vi "Corr_coeff_array.vi"(2 "Sampling frequency":dbl format="%.2f", 3 "U2":dbl[](array[numeric]) format="%.2f", 4 "U1":dbl[](array[numeric]) format="%.2f", 5 "Slippage range":i32) -> (0 "Correlation Coefficient":dbl[](array[numeric]) format="%.2f", 1 "Time":dbl[](array[numeric]) format="%.2f")   [LabVIEW 2010]
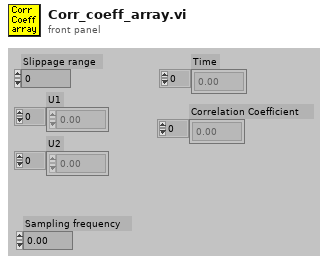
[diagram p1: front panel]
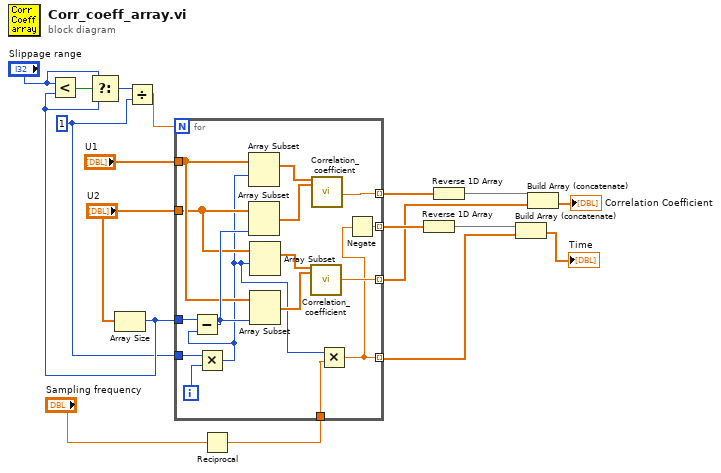
[diagram p0: block diagram]
diagram:
  w1 = 1 ("y")
  n1 = Array Size(array="U2") -> (size(s)=w7:i32)
  n2 = Less?(x="Slippage range", y=w7) -> (x < y?=w8:bool)
  n3 = Select(t="Slippage range", s=w8, f=w7) -> (s? t:f=w3:i32)
  n4 = Divide(x=w3, y=w1) -> (x/y=w2:dbl)
  n5 = Reciprocal(x="Sampling frequency") -> (1/x=w18:dbl)
  n6 = for {
    N: w2 -> [_]
    tunnel: w7 -> [w34]
    tunnel: "U1" -> [w28]
    tunnel: "U2" -> [w27]
    tunnel: [w26] -> w13 mode=indexing
    tunnel: [w25] -> w14 mode=indexing
    tunnel: w18 -> [w24]
    tunnel: [w23] -> w15 mode=indexing
    tunnel: [w22] -> w5 mode=indexing
    tunnel: w1 -> [w21]
    i -> [w20]
    n7 = Multiply(x=w21, y=w20) -> (x*y=w19:i32)
    n8 = Subtract(x=w34, y=w19) -> (x-y=w29:i32)
    n9 = Array Subset(array=w28, index=w19) -> (w33:dbl[])  [unwired: 1 in]
    n10 = Array Subset(array=w27, length=w29) -> (w32:dbl[])  [unwired: 1 in]
    n11 = Array Subset(array=w27, index=w19) -> (w30:dbl[])  [unwired: 1 in]
    n12 = Array Subset(array=w28, length=w29) -> (w31:dbl[])  [unwired: 1 in]
    n13 = call "Correlation_coefficient.vi"("U"=w30, "W"=w31) -> ("Correlation coefficient"=w25:dbl)  [unwired: 17 in]
    n14 = call "Correlation_coefficient.vi"("U"=w33, "W"=w32) -> ("Correlation coefficient"=w26:dbl)  [unwired: 17 in]
    n15 = Multiply(x=w19, y=w24) -> (x*y=w22:dbl)
    n16 = Negate(x=w22) -> (-x=w23:dbl)
  }
  n17 = Reverse 1D Array(array=w15) -> (reversed array=w6:dbl[])
  n18 = Reverse 1D Array(array=w13) -> (reversed array=w4:dbl[])
  n19 = Build Array (concatenate)(w6, w5) -> (→"Time":dbl[])
  n20 = Build Array (concatenate)(w4, w14) -> (→"Correlation Coefficient":dbl[])
